vi "load_profile.vi"(8 "error in (no error)":errorcluster, 11 "Path":path) -> (0 "error out":errorcluster, 3 "Array":T1[](array[typedef]) {"torque" format="%.1f"})   [LabVIEW 2019]
uses:
  core_setup.ctl
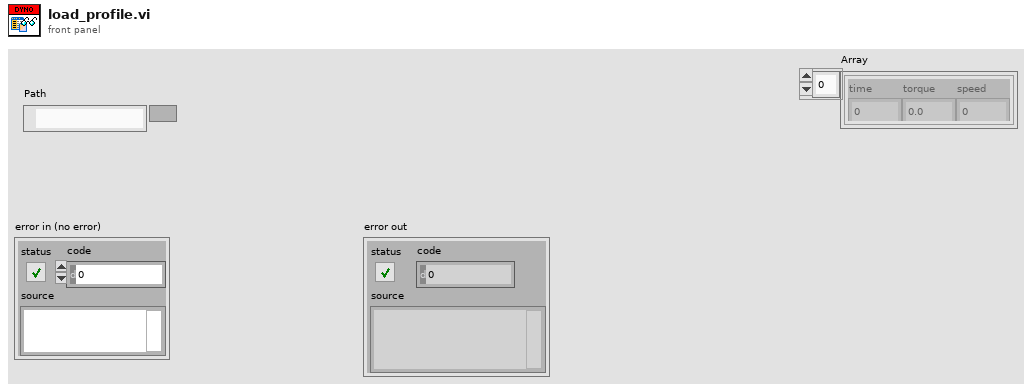
[diagram p1: front panel]
types:
  T1 = typedef "core_setup.ctl" = cluster{"time":i32, "torque":dbl, "speed":i32}
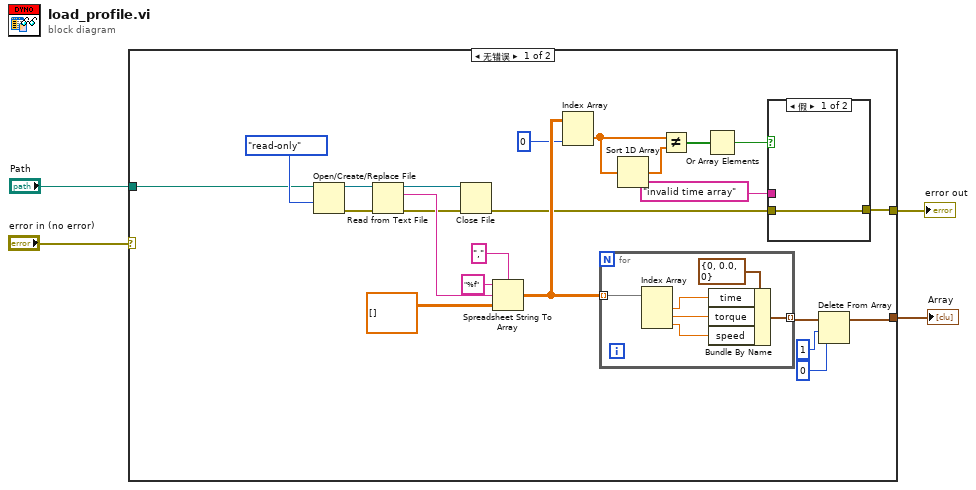
[diagram p0: block diagram]
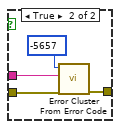
[diagram p2: hidden frame]
diagram:
  n1 = case shown="无错误" "error in (no error)" {
    selector: "error in (no error)" -> [_ w39]
    tunnel: "Path" -> [w18 _]
    tunnel: [w7 _] -> w3
    tunnel: [w10 w39] -> w2
    frame No Error {
      n2 = Open/Create/Replace File(file path (use dialog)=w18, access (0:read/write)=enum16{"read/write", "read-only", "write-only"}."read-only") -> (refnum out=w26:refnum<file>, error out=w25:errorcluster)  [unwired: 4 in, 1 out]
      n3 = Read from Text File(file (use dialog)=w26, error in=w25) -> (refnum out=w23:refnum<file>, text=w24:string, error out=w22:errorcluster)  [unwired: 2 in, 1 out]
      n4 = Close File(refnum=w23, error in=w22) -> (error out=w11:errorcluster)  [unwired: 1 out]
      n5 = Spreadsheet String To Array(delimiter (Tab)=",", format string="%f", spreadsheet string=w24, array type (2D Dbl)=dbl[][] []) -> (array=w17:dbl[][])
      n6 = Index Array(array=w17, index (col)=0 ("disabled index (col)")) -> (element=w15:dbl[])  [unwired: 1 in]
      n7 = for {
        tunnel: w17 -> [w38] mode=indexing
        tunnel: [w33] -> w8 mode=indexing
        n8 = Index Array(array=w38) -> (element #1=w36:dbl, element #2=w35:dbl, element #3=w34:dbl)  [unwired: 3 in]
        n9 = Bundle By Name(cluster=T1 {"time"=0, "torque"=0.0, "speed"=0} ("Cluster"), "time"=w36, "torque"=w35, "speed"=w34) -> (w33:T1)
      }
      n10 = Sort 1D Array(array=w15) -> (sorted array=w14:dbl[])
      n11 = Not Equal?(x=w15, y=w14) -> (x != y?=w13:bool[])
      n12 = Or Array Elements(Boolean array=w13) -> (logical OR=w12:bool)
      n13 = case shown="假" w12 {
        tunnel: w11 -> [w28 w32]
        tunnel: [w28 w31] -> w10
        tunnel: "invalid time array" ("delimiter (Tab)") -> [_ w30]
        frame False {
        }
        frame True {
          n14 = call <vilib>:"Error Cluster From Error Code.vi"("error in (no error)"=w32, "error message (\"\")"=w30, "error code (0)"=-5657) -> ("error out"=w31:errorcluster)  [unwired: 6 in]
        }
      }
      n15 = Delete From Array(array=w8, length=1 ("长度"), index=0 ("索引")) -> (array with subset deleted=w7:T1[])  [unwired: 1 out]
    }
    frame Error {
    }
  }
  "error out" <- w2
  "Array" <- w3
